vi "Insert VI in Subpanel.vi"(0 "VI Ref":refnum<vi>, 2 "Parent":refnum<vi>, 7 "SubPanel":refnum<vi>, 9 "inputs":cluster{"name":string, "value":variant}[](array[cluster]), 11 "error in (no error)":errorcluster, 12 "close event":bool) -> (8 "close event":refnum<user-event>, 15 "error out":errorcluster)   [LabVIEW 2020]
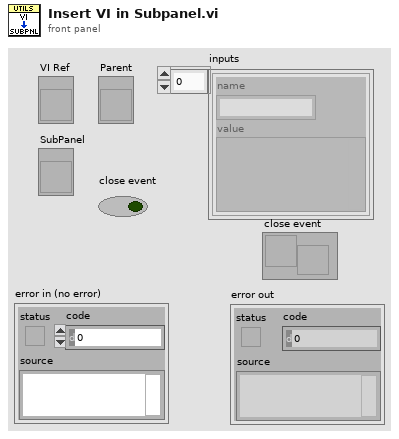
[diagram p1: front panel]
types:
  T1 = enum16{"Always On", "Always Off", "Off While Running"}
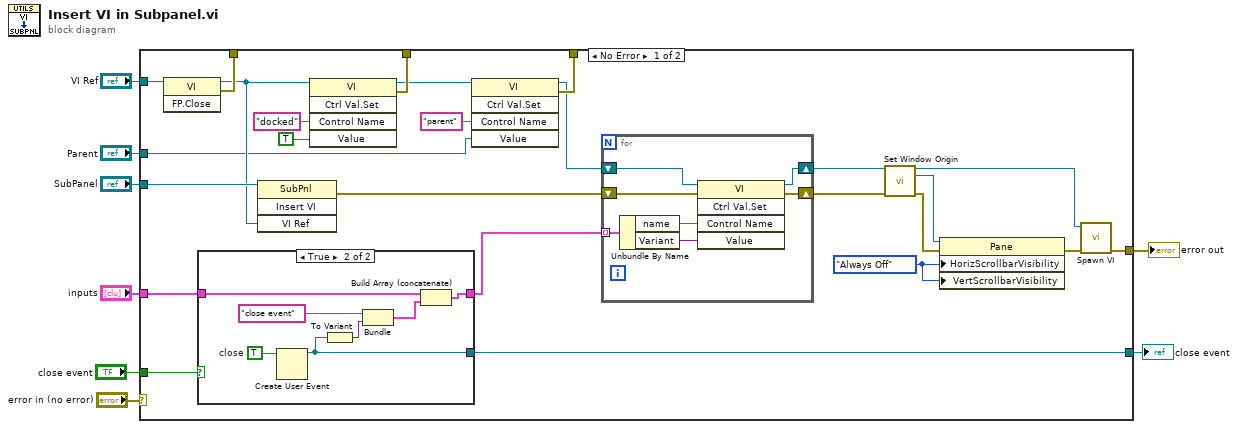
[diagram p0: block diagram]
diagram:
  n1 = case shown="No Error" "error in (no error)" {
    selector: "error in (no error)" -> [_ w49]
    tunnel: [w27 w49] -> w7
    tunnel: "SubPanel" -> [w32 _]
    tunnel: "VI Ref" -> [w26 _]
    tunnel: [w31 _] -> _
    tunnel: [w25 _] -> _
    tunnel: [w21 _] -> _
    tunnel: "Parent" -> [w20 _]
    tunnel: "inputs" -> [w11 _]
    tunnel: "close event" -> [w12 _]
    tunnel: [w9 _] -> w1
    frame No Error {
      w33 = T1."Always Off" ("Horizontal Scrollbar Visibility")
      n2 = invoke class="VI" method="FP.Close"(reference=w26) -> (reference out=w24:refnum<vi>, error out=w31:errorcluster)  [unwired: 2 in, 1 out]
      n3 = case shown="True" w12 {
        tunnel: w11 -> [w34 w41]
        tunnel: [w34 w36] -> w10
        tunnel: [_ w39] -> w9
        frame False {
        }
        frame True {
          w40 = TRUE  # close
          n4 = Create User Event(user event datatype=w40) -> (user event=w39:refnum<user-event>)  [unwired: 1 in, 1 out]
          n5 = To Variant(anything=w39) -> (Variant=w37:variant)
          n6 = Bundle("close event", "Variant"=w37) -> (w35:cluster{string, "Variant":variant})  [unwired: 1 in]
          n7 = Build Array (concatenate)(w41, w35) -> (w36:cluster{"name":string, "Variant":variant}[])
        }
      }
      n8 = invoke on="Invoke Node" class="SubPnl" method="Insert VI"(reference=w32, "VI Ref"=w24) -> (error out=w16:errorcluster)  [unwired: 2 in, 3 out]
      n9 = invoke class="VI" method="Ctrl Val.Set"(reference=w24, "Control Name"="docked", "Value"=TRUE) -> (reference out=w22:refnum<vi>, error out=w25:errorcluster)  [unwired: 2 in, 3 out]
      n10 = invoke class="VI" method="Ctrl Val.Set"(reference=w22, "Control Name"="parent", "Value"=w20) -> (reference out=w15:refnum<vi>, error out=w21:errorcluster)  [unwired: 2 in, 3 out]
      n11 = for {
        shift-right: [w45] -> w13
        shift-left: w16 -> [w48]
        shift-right: [w46] -> w14
        shift-left: w15 -> [w47]
        tunnel: w10 -> [w44] mode=indexing
        n12 = Unbundle By Name(w44) -> ("name"=w43:string, "Variant"=w42:variant)
        n13 = invoke class="VI" method="Ctrl Val.Set"(reference=w47, error in=w48, "Control Name"=w43, "Value"=w42) -> (reference out=w46:refnum<vi>, error out=w45:errorcluster)  [unwired: 1 in, 3 out]
      }
      n14 = call "Set Window Origin.vi"("VI in"=w14, "error in (no error)"=w13) -> ("VI out"=w17:refnum<vi>, "pane"=w19:refnum<vi>, "error out"=w18:errorcluster)  [unwired: 11 in]
      n15 = property class="Pane"(reference=w19, error in=w18, "HorizScrollbarVisibility"=w33, "VertScrollbarVisibility"=w33) -> (error out=w28:errorcluster)  [unwired: 1 out]
      n16 = call "Spawn VI.vi"("error in (no error)"=w28, "VI reference"=w17) -> ("error out"=w27:errorcluster)  [unwired: 8 in, 1 out]
    }
    frame Error {
    }
  }
  "error out" <- w7
  "close event" <- w1
